vi "数据库存储.vi"(2 "输出簇 2":T1) -> ()   [LabVIEW 2010]
panel:
  in  "error in (no error)":errorcluster caption="错误输入（无错误）"
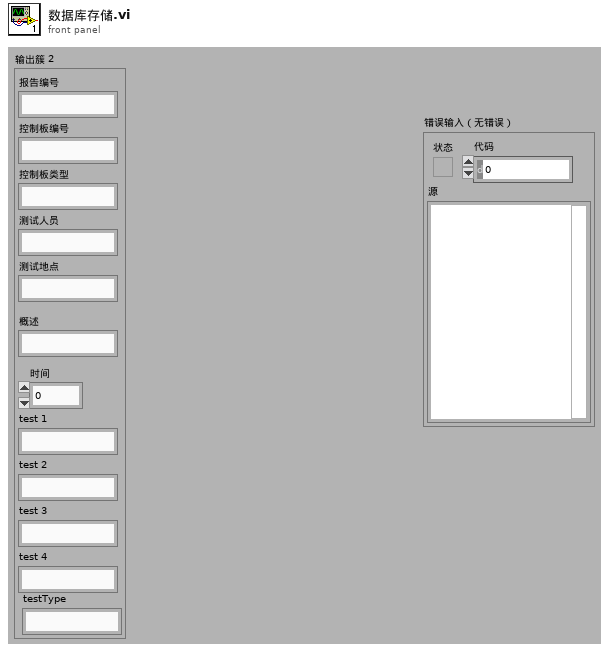
[diagram p1: front panel]
types:
  T1 = cluster{"报告编号":string, "控制板编号":string, "控制板类型":string, "测试人员":string, "测试地点":string, "概述":string, "时间":u64, "test 1":string, "test 2":string, "test 3":string, "test 4":string, "testType":string}
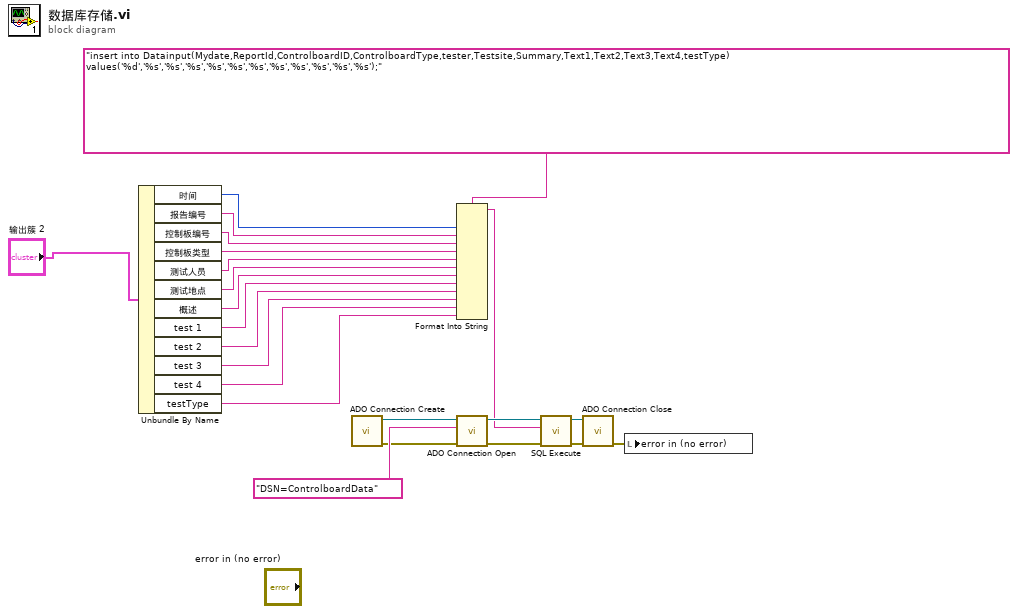
[diagram p0: block diagram]
diagram:
  n1 = Unbundle By Name("输出簇 2") -> ("时间"=w13:u64, "报告编号"=w12:string, "控制板编号"=w11:string, "控制板类型"=w10:string, "测试人员"=w9:string, "测试地点"=w8:string, "概述"=w7:string, "test 1"=w6:string, "test 2"=w5:string, "test 3"=w4:string, "test 4"=w3:string, "testType"=w1:string)
  n2 = call "ADO Connection Create.vi"() -> ("error out"=w16:errorcluster, "ADODB._Connection Out"=w15:refnum<k7>)  [unwired: 10 in]
  n3 = Format Into String(format string="insert into Datainput(Mydate,ReportId,ControlboardID,ControlboardType,tester,Testsite,Summary,Text1,Text2,Text3,Text4,testType) values('%d','%s','%s','%s','%s','%s','%s','%s','%s','%s','%s','%s');", w13, w12, w11, w10, w9, w8, w7, w6, w5, w4, w3, w1) -> (resulting string=w14:string)  [unwired: 2 in, 1 out]
  n4 = call "ADO Connection Open.vi"("error in (no error)"=w16, "ConnectionString"="DSN=ControlboardData", "ADODB._Connection In"=w15) -> ("error out"=w19:errorcluster, "ADODB._Connection Out"=w22:refnum<k7>)  [unwired: 7 in]
  n5 = call "SQL Execute.vi"("error in (no error)"=w19, "Command Text"=w14, "ADODB._Connection In"=w22) -> ("error out"=w18:errorcluster, "ADODB._Connection Out"=w21:refnum<k7>)  [unwired: 5 in, 2 out]
  n6 = call "ADO Connection Close.vi"("error in (no error)"=w18, "ADODB._Connection In"=w21) -> ("error out"=w17:errorcluster)  [unwired: 8 in, 1 out]
  n7 = local write "error in (no error)"(w17) -> ()
